vi "reward_behavior_michelle_visjitter_conswinAdapt_enticefx_TSLog_VF_fortraining_lightdetectionOG.vi"() -> ()   [LabVIEW 2019]
doc: "The myRIO Project template acquires acceleration data from the onboard accelerometer and displays the changes of acceleration values in a waveform chart."
uses:
  <vilib>/Analysis/Matrix/Datatypes/RealMatrix.ctl
  <vilib>/myRIO/Instrument Drivers/Onboard IO/DIO/typedefs/DIO Reference.ctl
  <vilib>/myRIO/Common/Instrument Driver Framework/Utilities/typedefs/myRIO Generic Hardware Reference.ctl
  <vilib>/myRIO/Common/Instrument Driver Framework/Utilities/typedefs/Hardware Version Enum.ctl
  <vilib>/myRIO/Common/Instrument Driver Framework/Utilities/typedefs/myRIO v1.0 Reference.ctl
  <vilib>/myRIO/Common/Instrument Driver Framework/Utilities/typedefs/Generic FPGA Reference.ctl
  <vilib>/myRIO/Common/Instrument Driver Framework/myRIO v1.0/DIO/typedefs/DIO Channels List.ctl
  <vilib>/myRIO/Common/Instrument Driver Framework/myRIO v1.0/DIO/typedefs/DIO Channels Enum.ctl
  <vilib>/userdefined/High Color/nirio_resource_hc.ctl
  <vilib>/myRIO/Common/Instrument Driver Framework/myRIO v1.0/Encoder/typedefs/Encoder Signal Mode.ctl
  <vilib>/myRIO/Instrument Drivers/Onboard IO/Encoder/typedefs/Encoder Reference.ctl
  <vilib>/myRIO/Common/Instrument Driver Framework/myRIO v1.0/Encoder/typedefs/Encoder Channels Enum.ctl
  <vilib>/myRIO/Common/Instrument Driver Framework/myRIO v1.0/Encoder/typedefs/Encoder Configuration v1.0.ctl
  <vilib>/myRIO/Instrument Drivers/Onboard IO/AI/typedefs/AI Reference.ctl
  <vilib>/myRIO/Common/Instrument Driver Framework/myRIO v1.0/AI/typedefs/AI Channels List.ctl
  <vilib>/myRIO/Common/Instrument Driver Framework/myRIO v1.0/AI/typedefs/AI Channels Enum.ctl
  <vilib>/myRIO/Common/Instrument Driver Framework/Utilities/typedefs/Analog Scaling Constants List.ctl
  <vilib>/myRIO/Common/Instrument Driver Framework/Utilities/typedefs/Analog Scaling Constants.ctl
  <vilib>/myRIO/Common/Instrument Driver Framework/Utilities/vis/Is FPGA Ref Available.vi
  <vilib>/myRIO/Common/Instrument Driver Framework/myRIO v1.0/DIO/vis/myRIO v1.1 Open DIO.vi
  <vilib>/myRIO/Instrument Drivers/Onboard IO/DIO/vis/Write.vi
  <vilib>/myRIO/Common/Instrument Driver Framework/myRIO v1.0/Encoder/vis/myRIO v1.1 Open Encoder.vi
  <vilib>/myRIO/Instrument Drivers/Onboard IO/Encoder/vis/Read.vi
  <vilib>/myRIO/Common/Instrument Driver Framework/myRIO v1.0/AI/vis/myRIO v1.1 Open AI.vi
  <vilib>/myRIO/Instrument Drivers/Onboard IO/AI/vis/Read.vi
  <vilib>/myRIO/Instrument Drivers/Onboard IO/DIO/vis/Read.vi
  <vilib>/myRIO/Common/Instrument Driver Framework/Utilities/vis/Validate Channels.vi
  <vilib>/myRIO/Common/Instrument Driver Framework/myRIO v1.0/DIO/vis/myRIO v1.0 Reserve DIO.vi
  <vilib>/myRIO/Common/Instrument Driver Framework/myRIO v1.0/Encoder/vis/myRIO v1.0 Reserve Encoder.vi
  <vilib>/myRIO/Common/Instrument Driver Framework/myRIO v1.0/AI/vis/myRIO v1.0 Reserve AI.vi
  <vilib>/myRIO/Common/Instrument Driver Framework/myRIO v1.0/Resource Manager/vis/myRIO v1.0 Reserve Channel List.vi
  <vilib>/myRIO/Common/Instrument Driver Framework/myRIO v1.0/DIO/vis/myRIO v1.0 Build MUX Configuration DIO.vi
  <vilib>/myRIO/Common/Instrument Driver Framework/myRIO v1.0/Encoder/vis/myRIO v1.0 Build MUX Configuration Encoder.vi
  <vilib>/myRIO/Common/Instrument Driver Framework/myRIO v1.0/AI/vis/myRIO v1.0 Build MUX Configuration AI.vi
  <vilib>/myRIO/Common/Instrument Driver Framework/myRIO v1.0/Resource Manager/vis/myRIO v1.0 Reserve Channel.vi
  <vilib>/myRIO/Common/Instrument Driver Framework/myRIO v1.0/Resource Manager/vis/myRIO v1.0 Unreserve Channel.vi
  <vilib>/myRIO/Common/Instrument Driver Framework/myRIO v1.0/Resource Manager/vis/myRIO v1.0 Create Configuration List.vi
  <vilib>/myRIO/Common/Instrument Driver Framework/myRIO v1.0/Resource Manager/vis/myRIO v1.0 Build Mutex Name.vi
  <vilib>/Utility/VariantDataType/GetNumericInfo.vi
  <vilib>/Utility/error.llb/Error Cluster From Error Code.vi
  <vilib>/myRIO/Common/Instrument Driver Framework/myRIO v1.0/myRIO v1.1 Open.vi
  <vilib>/myRIO/Common/Instrument Driver Framework/Utilities/vis/IO Manager.vi
  <vilib>/myRIO/Common/Instrument Driver Framework/Utilities/vis/Configuration Manager.vi
  <vilib>/myRIO/Common/Instrument Driver Framework/myRIO v1.0/Resource Manager/vis/myRIO v1.0 Configure IO.vi
  <vilib>/myRIO/Common/Instrument Driver Framework/myRIO v1.0/myRIO v1.0 Close.vi
  <vilib>/myRIO/Common/Instrument Driver Framework/myRIO v1.0/Encoder/vis/myRIO v1.0 Configure Encoder.vi
  <vilib>/myRIO/Common/Instrument Driver Framework/myRIO v1.0/Encoder/vis/myRIO v1.0 Read Encoder.vi
  <vilib>/myRIO/Common/Instrument Driver Framework/myRIO v1.0/DIO/vis/myRIO v1.0 Write DIO.vi
  <vilib>/myRIO/Common/Instrument Driver Framework/myRIO v1.0/DIO/vis/myRIO v1.0 Read DIO.vi
  <vilib>/myRIO/Common/Instrument Driver Framework/myRIO v1.0/AI/vis/myRIO v1.0 Get Scaling Constants AI.vi
  <vilib>/myRIO/Common/Instrument Driver Framework/myRIO v1.0/AI/vis/myRIO v1.0 Read AI.vi
  <vilib>/myRIO/Express VI/Onboard IO/Encoder/Encoder Express VI.xnode
  <vilib>/myRIO/Instrument Drivers/Onboard IO/Encoder/vis/myRIO Encoder Open.xnode
  <vilib>/myRIO/Common/Instrument Driver Framework/myRIO v1.0/Encoder/typedefs/Encoder Count Direction Enum.ctl
  <vilib>/myRIO/Express VI/Onboard IO/DO/DO Express VI.xnode
  <vilib>/myRIO/Instrument Drivers/Onboard IO/DIO/vis/myRIO DIO Open.xnode
  <vilib>/myRIO/Express VI/Onboard IO/DI/DI Express VI.xnode
  <vilib>/myRIO/Express VI/Onboard IO/AI/AI Express VI.xnode
  <vilib>/myRIO/Instrument Drivers/Onboard IO/AI/vis/myRIO AI Open.xnode
  <vilib>/myRIO/Instrument Drivers/Onboard IO/Encoder/Encoder.lvlib
  <vilib>/myRIO/Instrument Drivers/Onboard IO/DIO/DIO.lvlib
  <vilib>/myRIO/Instrument Drivers/Onboard IO/AI/AI.lvlib
  <vilib>/Analysis/Matrix/NI_Matrix.lvlib
panel:
  out "Light":dbl
  out "LightPlot":dbl[](graph)
  out "LightArray":dbl[](array[numeric])
  out "AutoEnticeLimit":i32=1000
  out "GetVidFrame":i32
  out "VidTS":dbl[][](array[numeric])
  out "VidFrameClock":i32
  out "EntTS":dbl[][](array[numeric])
  out "TimeLag":dbl
  out "Lag2":dbl
  out "TestTime":dbl
  out "RewTS":dbl[][](array[numeric])
  out "ConsTS":dbl[][](array[numeric])
  out "LickTS":dbl[][](array[numeric])
  out "ContrastChoice":dbl
  out "Its":i32
  out "BurstCriteria":dbl
  out "LickBurst 2":bool
  out "LickBurst":bool
  out "Enticements":i32
  in  "Entice":bool
  out "Misses":i32
  out "GoAhead":bool
  out "TimeOutDuration":i32
  out "ActiveTime":dbl
  out "ConsumptionGo":bool=TRUE
  out "Consumption_Period":i32
  out "Watch_Display":bool=TRUE
  in  "Give reward":bool
  out "Timings":dbl[](array[numeric])
  out "ISI":dbl
  out "ISI start time":dbl
  out "Time_out":bool=TRUE
  out "Time since lick":dbl
  out "Time of last lick":dbl
  out "Rewarded trials":dbl[](array[numeric])
  out "Rewards":u16
  out "Active Trial":bool
  out "Array temp2":T1
  out "Stimuli Loaded":bool
  out "Stim_ID":dbl[](array[numeric])
  out "Reward_mat":dbl[](array[numeric])
  out "Reward":bool=TRUE
  out "Frame clock":i32
  out "Licks":u32
  out "Lick":bool
  out "Time":dbl
  out "Stop":bool
  in  "Frames to collect":u32
  out "Overflow?":bool
  out "Counter Value":i32
  out "Velocity":dbl
  out "Velocity Plot":dbl[](graph)
  out "Velocity array":dbl[](array[numeric])
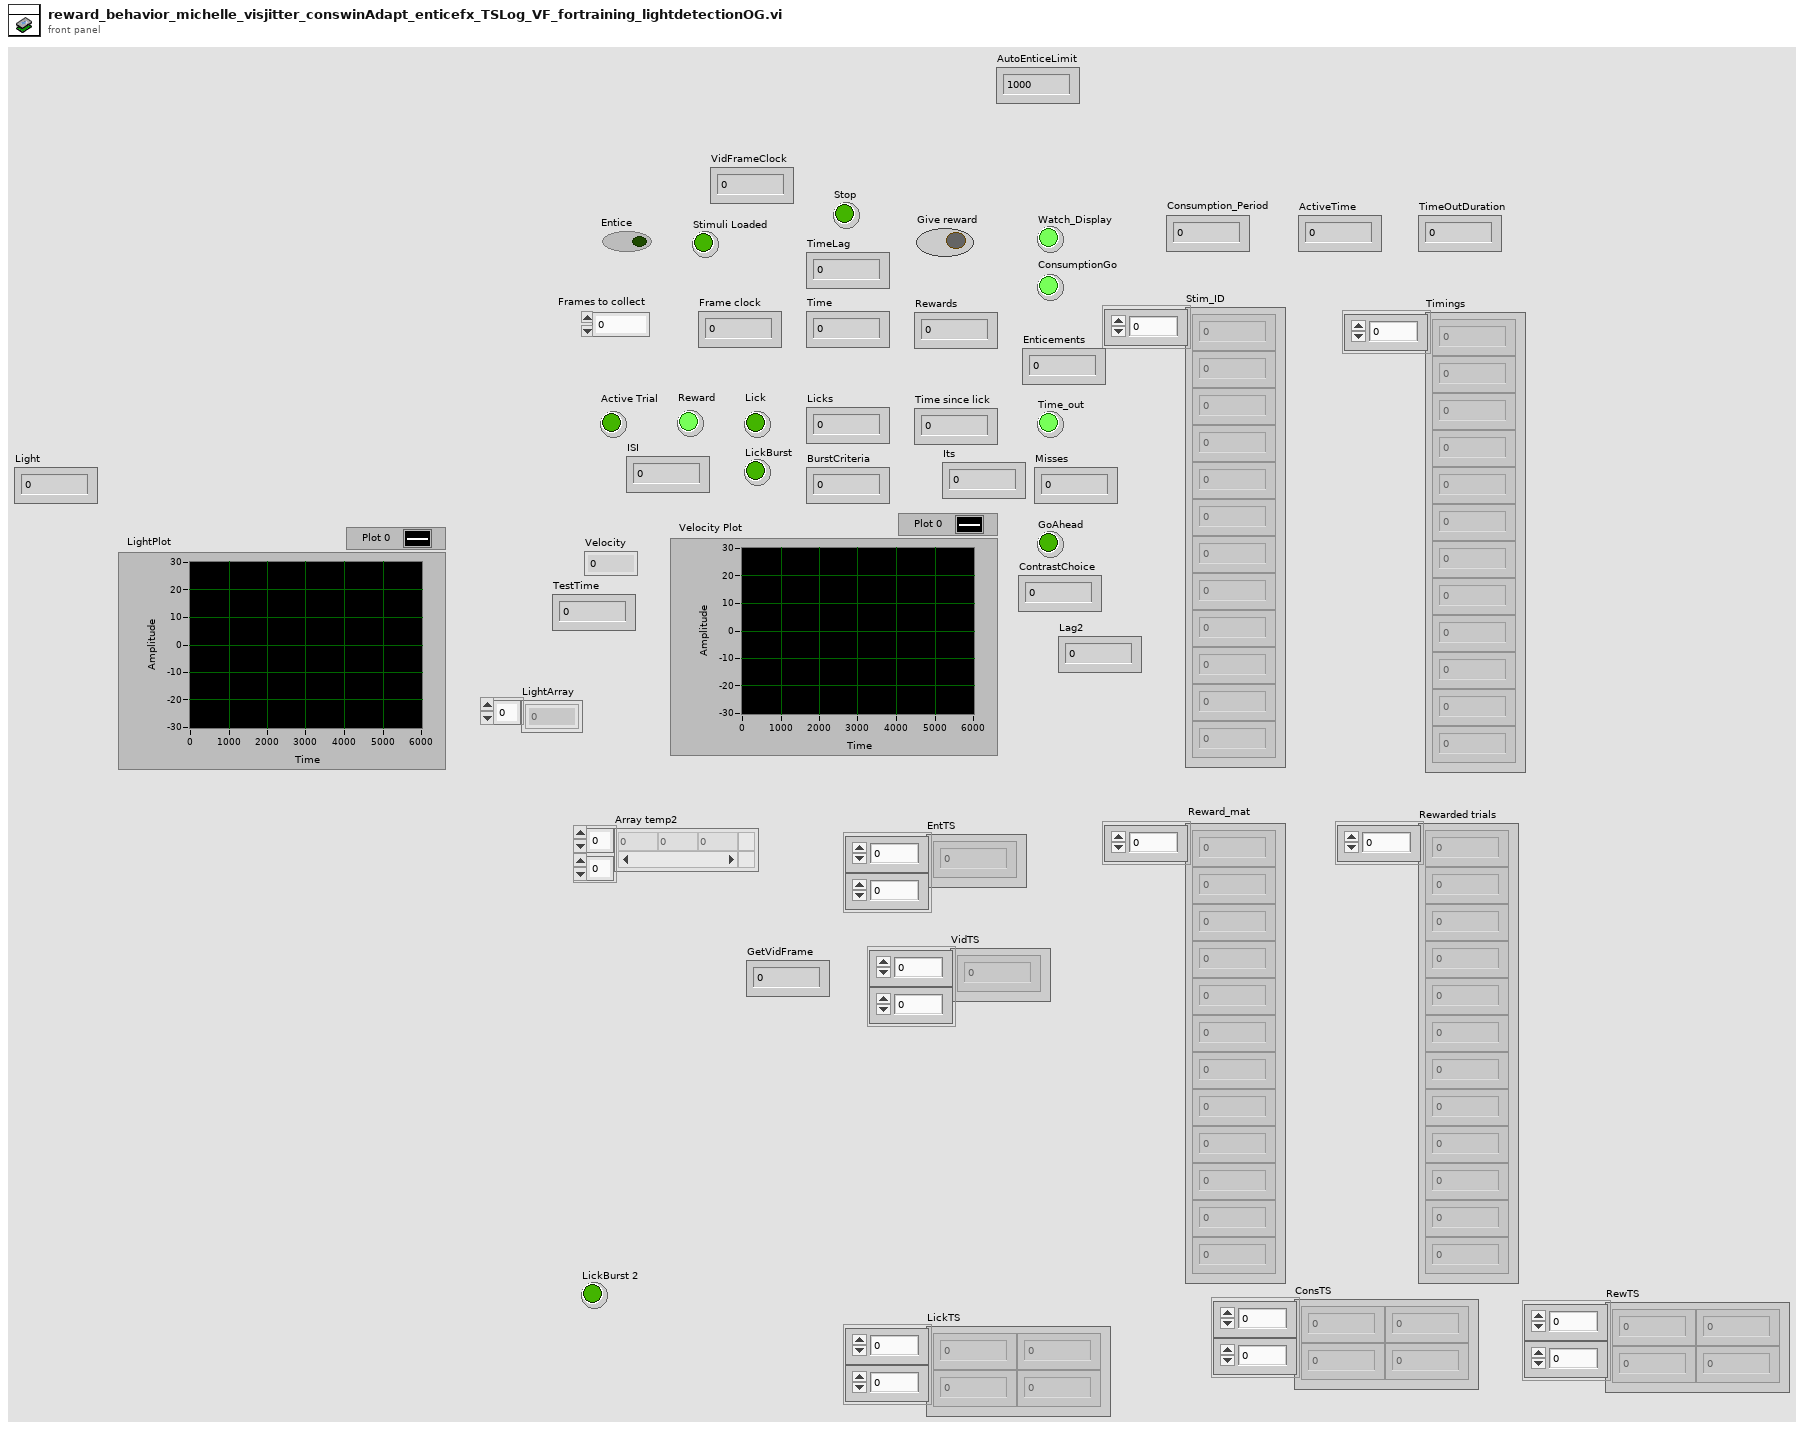
[diagram p1: front panel]
types:
  T1 = typedef "NI_Matrix.lvlib/RealMatrix.ctl" = dbl[][]
  T2 = typedef "DIO.lvlib/DIO Reference.ctl" = cluster{"myRIO Reference":T3, "DIO Channels List":T7}
  T3 = typedef "myRIO Generic Hardware Reference.ctl" = cluster{"myRIO Model":T4, "myRIO Hardware Reference":T5}
  T4 = typedef "Hardware Version Enum.ctl" = enum16{"Unknown", "myRIO-1900", "myRIO-1950", "roboRIO", "NI ELVIS RIO CM", "ELVIS III"}
  T5 = typedef "myRIO v1.0 Reference.ctl" = cluster{"Generic FPGA Reference":T6, "Allow multiple opens":bool}
  T6 = typedef "Generic FPGA Reference.ctl" = refnum<k20>
  T7 = typedef "DIO Channels List.ctl" = T8[]
  T8 = typedef "DIO Channels Enum.ctl" = enum16{"Not Connected", "C/DIO0", "C/DIO1", "C/DIO2", "C/DIO3", "C/DIO4", "C/DIO5", "C/DIO6", "C/DIO7", "A/DIO0", "A/DIO1", "A/DIO2", "A/DIO3", "A/DIO4", "A/DIO5", "A/DIO6", "A/DIO7", "A/DIO8", "A/DIO9", "A/DIO10", "A/DIO11", "A/DIO12", "A/DIO13", "A/DIO14", "A/DIO15", "A/DIO16", "A/DIO17", "A/DIO18", "A/DIO19", "B/DIO0", "B/DIO1", "B/DIO2", "B/DIO3", "B/DIO4", "B/DIO5", "B/DIO6", "B/DIO7", "B/DIO8", "B/DIO9", "B/DIO10", "B/DIO11", "B/DIO12", "B/DIO13", "B/DIO14", "B/DIO15", "B/DIO16", "B/DIO17", "B/DIO18", "B/DIO19", "LED0", "LED1", "LED2", "LED3", "Button0", "DIO/DIO0", "DIO/DIO1", "DIO/DIO2", "DIO/DIO3", "DIO/DIO4", "DIO/DIO5", "DIO/DIO6", "DIO/DIO7", "DIO/DIO8", "DIO/DIO9", "SPI/CS0", "SPI/CS1", "SPI/CS2", "SPI/CS3", "LED RADIO (Green)", "LED RADIO (Red)", "LED COMM (Green)", "LED COMM (Red)", "LED MODE (Green)", "LED MODE (Red)"}
  T9 = typedef "nirio_resource_hc.ctl" = tag
  T10 = typedef "Encoder.lvlib/Encoder Reference.ctl" = cluster{"myRIO Reference":T3, "Encoder Channels Enum":T11}
  T11 = typedef "Encoder Channels Enum.ctl" = enum16{"Not Connected", "C/ENC0", "C/ENC1", "A/ENC", "A/ENC0", "A/ENC1", "A/ENC2", "A/ENC3", "A/ENC4", "A/ENC5", "A/ENC6", "A/ENC7", "A/ENC8", "A/ENC9", "B/ENC", "B/ENC0", "B/ENC1", "B/ENC2", "B/ENC3", "B/ENC4", "B/ENC5", "B/ENC6", "B/ENC7", "B/ENC8", "B/ENC9", "DIO/ENC0", "DIO/ENC1", "DIO/ENC2", "DIO/ENC3", "DIO/ENC4"}
  T12 = typedef "Encoder Signal Mode.ctl" = enum16{"Quadrature phase signal", "Step and direction signal"}
  T13 = typedef "AI.lvlib/AI Reference.ctl" = cluster{"myRIO Reference":T3, "AI Channels List":T14, "AI Scaling Constants List":T16}
  T14 = typedef "AI Channels List.ctl" = T15[]
  T15 = typedef "AI Channels Enum.ctl" = enum16{"Not Connected", "AudioIn/Left", "AudioIn/Right", "C/AI0", "C/AI1", "A/AI0", "A/AI1", "A/AI2", "A/AI3", "A/AI4", "A/AI5", "A/AI6", "A/AI7", "B/AI0", "B/AI1", "B/AI2", "B/AI3", "B/AI4", "B/AI5", "B/AI6", "B/AI7", "AI/AI0", "AI/AI1", "AI/AI2", "AI/AI3", "A/AI0 (DIFF)", "A/AI1 (DIFF)", "A/AI2 (DIFF)", "A/AI3 (DIFF)", "B/AI0 (DIFF)", "B/AI1 (DIFF)", "B/AI2 (DIFF)", "B/AI3 (DIFF)"}
  T16 = typedef "Analog Scaling Constants List.ctl" = T17[]
  T17 = typedef "Analog Scaling Constants.ctl" = cluster{"LSB Weight (Volts)":dbl, "Offset (Volts)":dbl, "Signed?":bool}
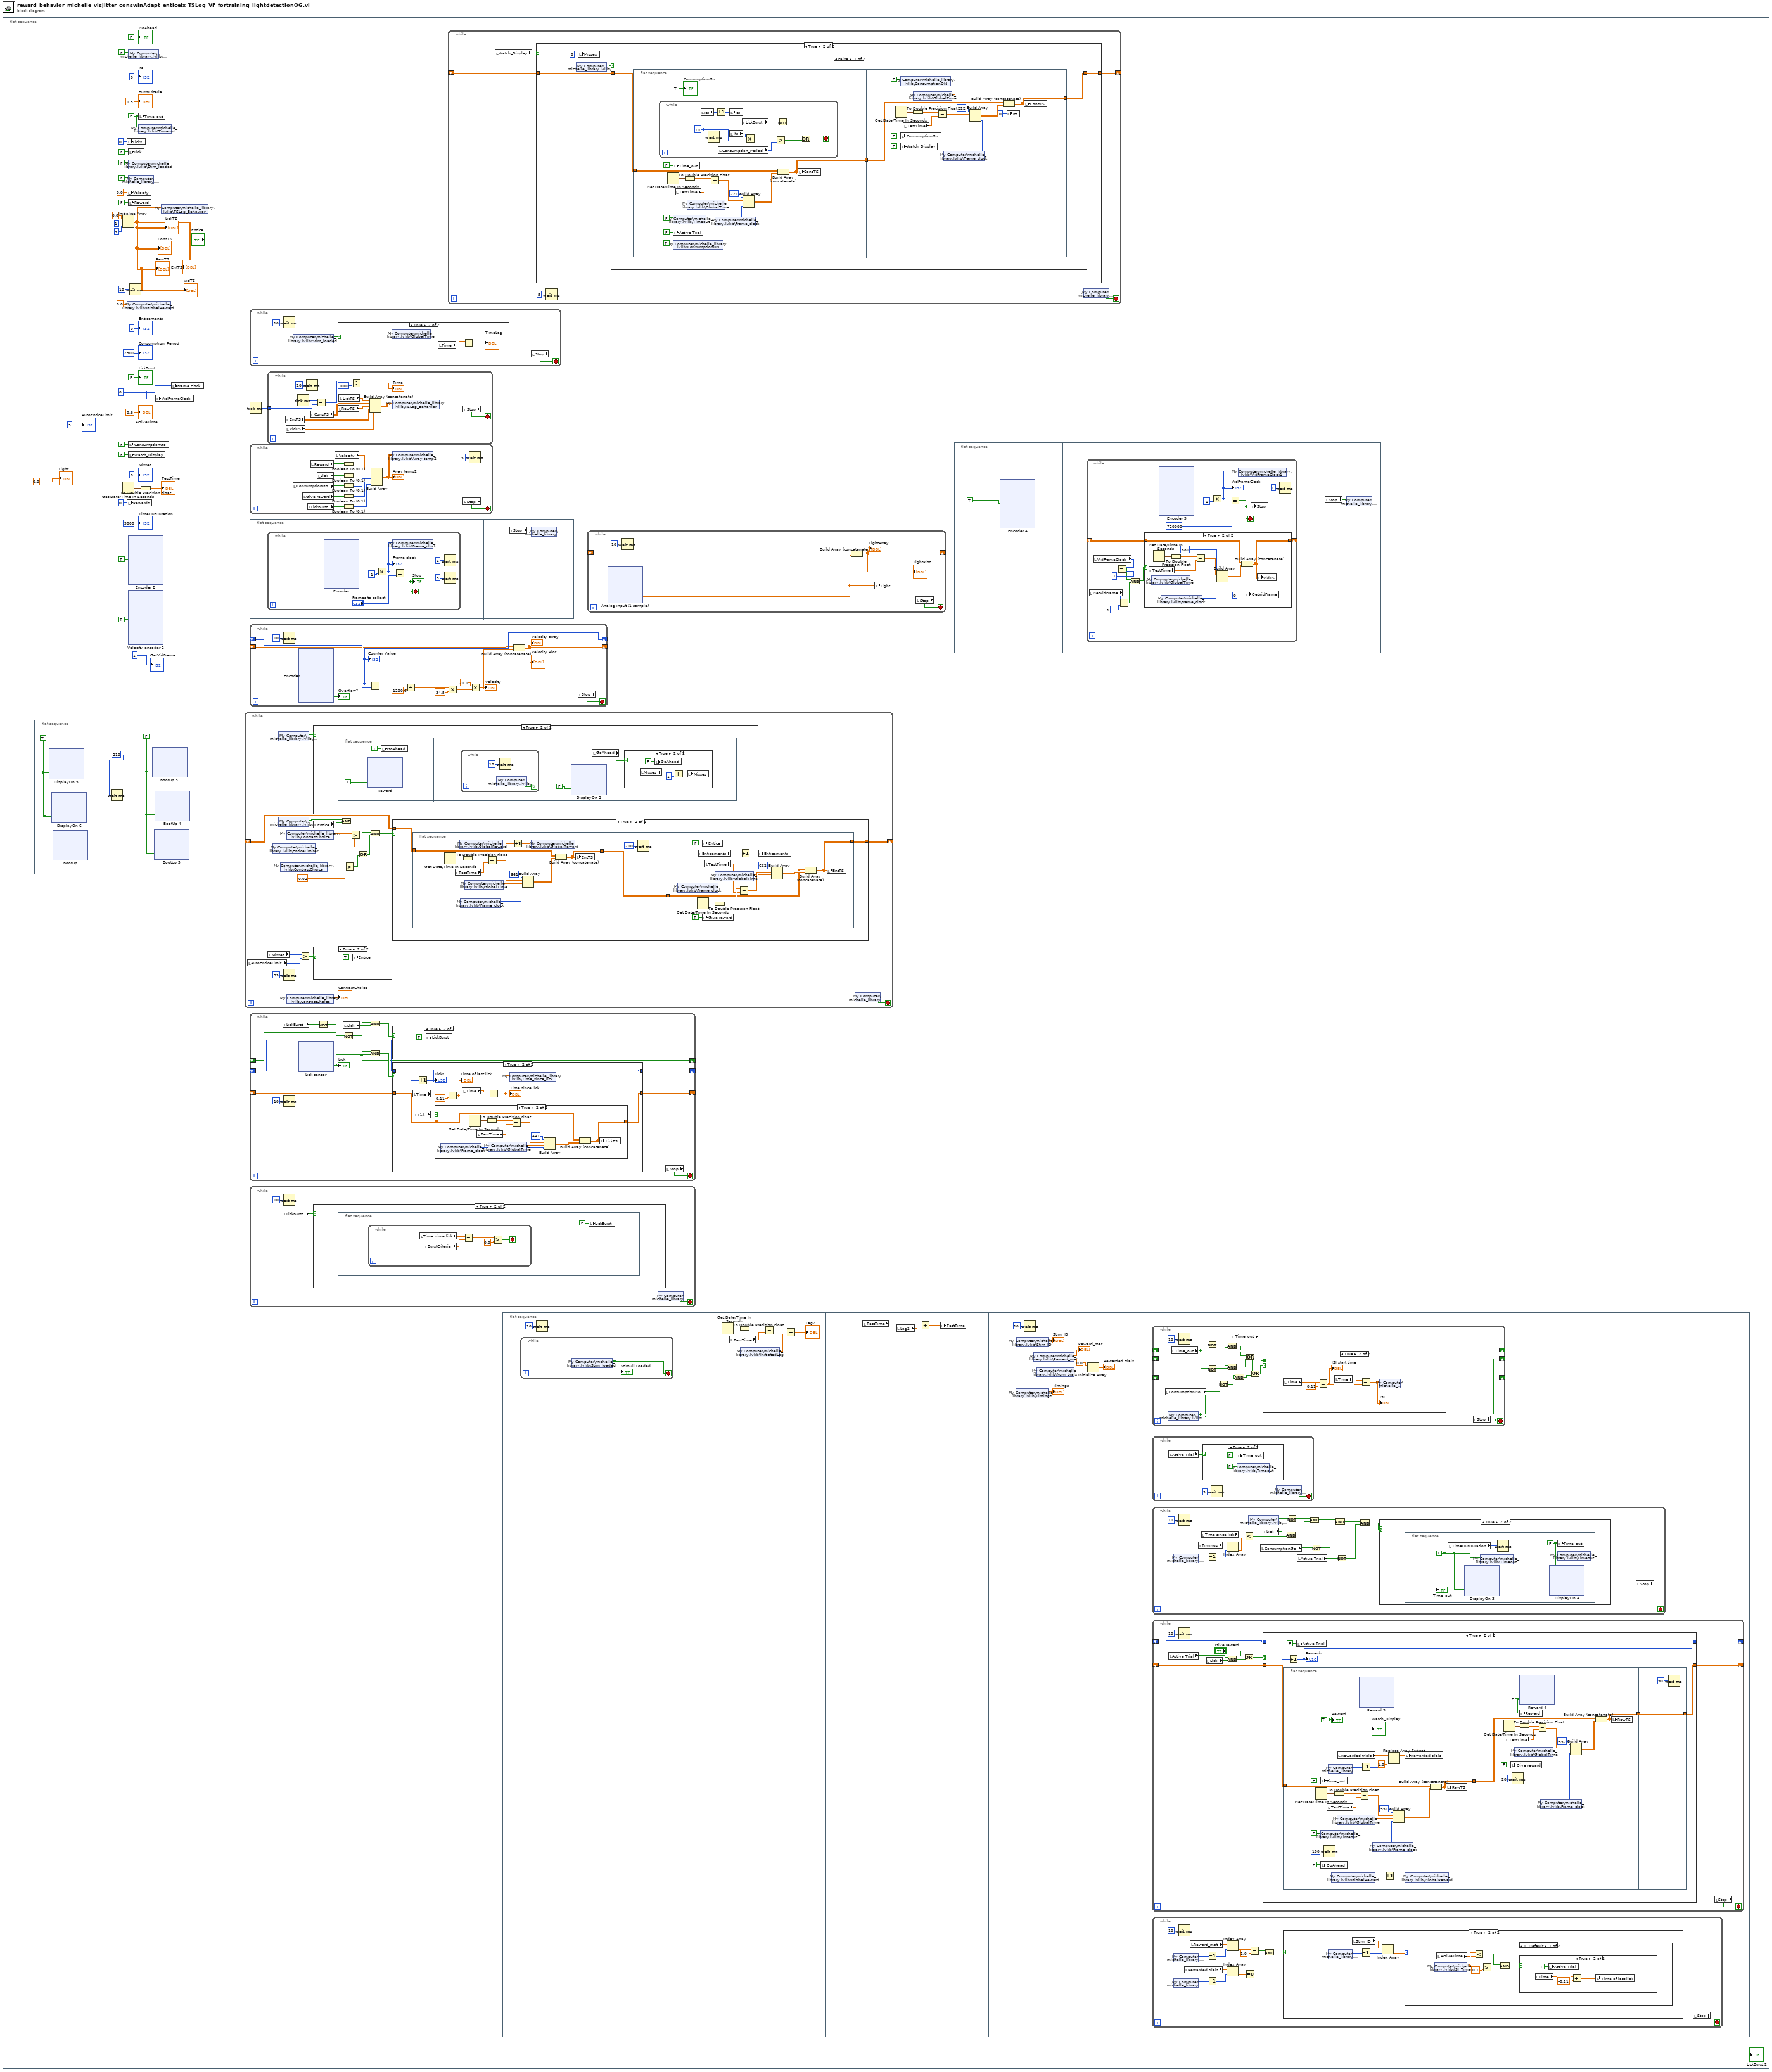
[diagram p0: block diagram]
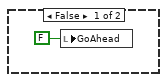
[diagram p7: hidden frame]
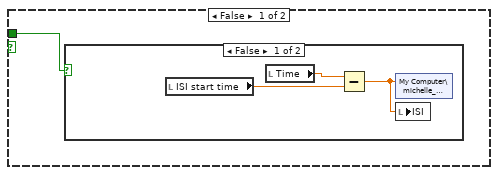
[diagram p13: hidden frame]
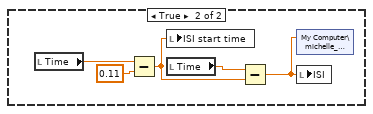
[diagram p14: hidden frame]
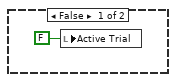
[diagram p15: hidden frame]
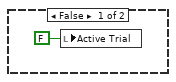
[diagram p16: hidden frame]
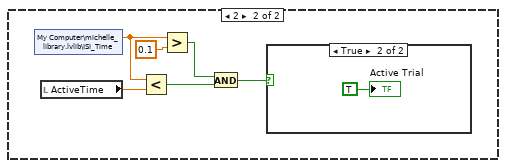
[diagram p17: hidden frame]
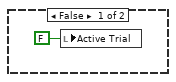
[diagram p18: hidden frame]
diagram:
  n1 = flat-sequence {
    frame #0 {
      w23 = FALSE ("Time_out")
      w5 = u32 0 ("Frames")
      n2 = flat-sequence {
        frame #0 {
          w35 = TRUE
          n3 = xnode "DisplayOn 5"("C/DIO2 (DIO2)"=w35) -> ()  [unwired: 1 in, 1 out]
          n4 = xnode "DisplayOn 6"("C/DIO1 (DIO1)"=w35) -> ()  [unwired: 1 in, 1 out]
          n5 = xnode "BootUp"("C/DIO3 (DIO3)"=w35) -> ()  [unwired: 1 in, 1 out]
        }
        frame #1 {
          n6 = Wait (ms)(milliseconds to wait=210) -> ()  [unwired: 1 out]
        }
        frame #2 {
          w142 = FALSE
          n7 = xnode "BootUp 3"("C/DIO2 (DIO2)"=w142) -> ()  [unwired: 1 in, 1 out]
          n8 = xnode "BootUp 5"("C/DIO3 (DIO3)"=w142) -> ()  [unwired: 1 in, 1 out]
          n9 = xnode "BootUp 4"("C/DIO1 (DIO1)"=w142) -> ()  [unwired: 1 in, 1 out]
        }
      }
      n10 = Get Date/Time In Seconds() -> (seconds since 1Jan1904=w7:timestamp)
      n11 = Initialize Array(0.0, 1, 3) -> (w4:dbl[][])
      "LickTS" <- w4
      "ConsTS" <- w4
      "RewTS" <- w4
      "EntTS" <- w4
      "VidTS" <- w4
      n12 = local write "Licks"(u32 0 ("Licks")) -> ()
      n13 = local write "Velocity"(0.0 ("Velocity")) -> ()
      n14 = shared-variable "My Computer\\michelle_library.lvlib\\GlobalReward"(0.0) -> ()  [unwired: 1 in, 1 out]
      n15 = local write "Rewards"(u16 0 ("Rewards")) -> ()
      n16 = shared-variable "My Computer\\michelle_library.lvlib\\Display"(FALSE ("Display")) -> ()  [unwired: 1 in, 1 out]
      n17 = local write "Lick"(FALSE ("Lick")) -> ()
      n18 = shared-variable "My Computer\\michelle_library.lvlib\\Stim_loaded"(FALSE ("Stim_loaded")) -> ()  [unwired: 1 in, 1 out]
      n19 = shared-variable "My Computer\\michelle_library.lvlib\\Stop"(FALSE ("Stop")) -> ()  [unwired: 1 in, 1 out]
      n20 = local write "Reward"(FALSE ("Give reward")) -> ()
      n21 = local write "ConsumptionGo"(FALSE ("ConsumptionGo")) -> ()
      n22 = local write "Watch_Display"(FALSE ("Watch_Display")) -> ()
      n23 = xnode "Encoder 2"("Reset Counter"=TRUE) -> ()  [unwired: 1 in, 4 out]
      n24 = xnode "Velocity encoder 2"("Reset Counter"=TRUE) -> ()  [unwired: 1 in, 4 out]
      n25 = Wait (ms)(milliseconds to wait=u32 10) -> ()  [unwired: 1 out]
      n26 = local write "Time_out"(w23) -> ()
      n27 = shared-variable "My Computer\\michelle_library.lvlib\\Timeout"(w23) -> ()  [unwired: 1 in, 1 out]
      n28 = To Double Precision Float(number=w7) -> (double precision float=→"TestTime":dbl)
      n29 = local write "VidFrameClock"(w5) -> ()
      n30 = shared-variable "My Computer\\michelle_library.lvlib\\TSLog_Behavior"(w4) -> ()  [unwired: 1 in, 1 out]
      n31 = local write "Frame clock"(w5) -> ()
      "Consumption_Period" <- 2500
      "ActiveTime" <- 0.6
      "TimeOutDuration" <- 3000
      "GoAhead" <- FALSE
      "Misses" <- 0
      "Enticements" <- 0
      "LickBurst" <- FALSE
      "BurstCriteria" <- 0.5
      "Its" <- 0
      "GetVidFrame" <- 1
      "AutoEnticeLimit" <- 5
      "Light" <- 0.0
    }
    frame #1 {
      n32 = while {
        shift-right: [w527] -> _
        shift-left: _ -> [w528]
        stop <- w538 stop-if-true
        n33 = local read "AutoEnticeLimit"() -> (w519:i32)
        n34 = local read "Misses"() -> (w520:i32)
        n35 = shared-variable "My Computer\\michelle_library.lvlib\\EnticeLimiter"() -> (w526:dbl)  [unwired: 1 in, 1 out]
        n36 = shared-variable "My Computer\\michelle_library.lvlib\\Display"() -> (w537:bool)  [unwired: 1 in, 1 out]
        n37 = shared-variable "My Computer\\michelle_library.lvlib\\Display"() -> (w535:bool)  [unwired: 1 in, 1 out]
        n38 = shared-variable "My Computer\\michelle_library.lvlib\\ContrastChoice"() -> (w522:dbl)  [unwired: 1 in, 1 out]
        n39 = Wait (ms)(milliseconds to wait=35) -> ()  [unwired: 1 out]
        n40 = shared-variable "My Computer\\michelle_library.lvlib\\ContrastChoice"() -> (w531:dbl)  [unwired: 1 in, 1 out]
        n41 = shared-variable "My Computer\\michelle_library.lvlib\\ContrastChoice"() -> (→"ContrastChoice":dbl)  [unwired: 1 in, 1 out]
        n42 = Greater?(x=w520, y=w519) -> (0:w536:bool)
        n43 = case shown="True" w537 {
          frame False {
            n44 = local write "GoAhead"(FALSE) -> ()
          }
          frame True {
            n45 = flat-sequence {
              frame #0 {
                n46 = xnode "Reward"("C/DIO2 (DIO2)"=TRUE) -> ()  [unwired: 1 in, 1 out]
                n47 = local write "GoAhead"(TRUE) -> ()
              }
              frame #1 {
                n48 = while {
                  stop <- w612 continue-if-true
                  n49 = shared-variable "My Computer\\michelle_library.lvlib\\Display"() -> (w612:bool)  [unwired: 1 in, 1 out]
                  n50 = Wait (ms)(milliseconds to wait=10) -> ()  [unwired: 1 out]
                }
              }
              frame #2 {
                n51 = xnode "DisplayOn 2"("C/DIO2 (DIO2)"=FALSE) -> ()  [unwired: 1 in, 1 out]
                n52 = local read "GoAhead"() -> (w614:bool)
                n53 = case shown="True" w614 {
                  frame False {
                  }
                  frame True {
                    n54 = local read "Misses"() -> (w653:i32)
                    n55 = local write "GoAhead"(FALSE) -> ()
                    n56 = Add(x=w653, y=1) -> (x+y=w651:i32)
                    n57 = local write "Misses"(w651) -> ()
                  }
                }
              }
            }
          }
        }
        n58 = local read "Entice"() -> (w534:bool)
        n59 = case shown="True" w536 {
          frame False {
          }
          frame True {
            n60 = local write "Entice"(TRUE) -> ()
          }
        }
        n61 = And(x=w535, y=w534) -> (x .and. y?=w532:bool)
        n62 = Greater?(x=w522, y=0.02) -> (0:w523:bool)
        n63 = Greater?(x=w531, y=w526) -> (0:w524:bool)
        n64 = Or(x=w524, y=w523) -> (x .or. y?=w525:bool)
        n65 = And(x=w532, y=w525) -> (x .and. y?=w530:bool)
        n66 = case shown="True" w530 {
          tunnel: w528 -> [w539 w543]
          tunnel: [w539 w540] -> w527
          frame False {
          }
          frame True {
            n67 = flat-sequence {
              tunnel: w543 -> [w546]
              tunnel: [w545] -> w542
              tunnel: w542 -> [w556]
              tunnel: [w556] -> w541
              tunnel: w541 -> [w560]
              tunnel: [w559] -> w540
              frame #0 {
                n68 = Get Date/Time In Seconds() -> (seconds since 1Jan1904=w553:timestamp)
                n69 = local read "TestTime"() -> (w548:dbl)
                n70 = shared-variable "My Computer\\michelle_library.lvlib\\GlobalReward"() -> (w555:dbl)  [unwired: 1 in, 1 out]
                n71 = shared-variable "My Computer\\michelle_library.lvlib\\Frame_clock"() -> (w544:u32)  [unwired: 1 in, 1 out]
                n72 = To Double Precision Float(number=w553) -> (double precision float=w552:dbl)
                n73 = shared-variable "My Computer\\michelle_library.lvlib\\GlobalTime"() -> (w547:dbl)  [unwired: 1 in, 1 out]
                n74 = Subtract(x=w552, y=w548) -> (x-y=w551:dbl)
                n75 = Increment(x=w555) -> (x+1=w554:dbl)
                n76 = Build Array(661, w551, w547, w544) -> (w550:T1)
                n77 = shared-variable "My Computer\\michelle_library.lvlib\\GlobalReward"(w554) -> ()  [unwired: 1 in, 1 out]
                n78 = Build Array (concatenate) ("Build Matrix")(w546, w550) -> (w545:T1)
                n79 = local write "EntTS"(w545) -> ()
              }
              frame #1 {
                n80 = Wait (ms)(milliseconds to wait=200) -> ()  [unwired: 1 out]
              }
              frame #2 {
                n81 = shared-variable "My Computer\\michelle_library.lvlib\\Frame_clock"() -> (w558:u32)  [unwired: 1 in, 1 out]
                n82 = Get Date/Time In Seconds() -> (seconds since 1Jan1904=w567:timestamp)
                n83 = local read "Enticements"() -> (w569:i32)
                n84 = local write "Entice"(FALSE) -> ()
                n85 = local write "Give reward"(TRUE) -> ()
                n86 = local read "TestTime"() -> (w561:dbl)
                n87 = To Double Precision Float(number=w567) -> (double precision float=w566:dbl)
                n88 = shared-variable "My Computer\\michelle_library.lvlib\\GlobalTime"() -> (w562:dbl)  [unwired: 1 in, 1 out]
                n89 = Subtract(x=w566, y=w561) -> (x-y=w565:dbl)
                n90 = Increment(x=w569) -> (x+1=w568:i32)
                n91 = local write "Enticements"(w568) -> ()
                n92 = Build Array(662, w565, w562, w558) -> (w564:T1)
                n93 = Build Array (concatenate) ("Build Matrix")(w560, w564) -> (w559:T1)
                n94 = local write "EntTS"(w559) -> ()
              }
            }
          }
        }
        n95 = shared-variable "My Computer\\michelle_library.lvlib\\Stop"() -> (w538:bool)  [unwired: 1 in, 1 out]
      }
      n96 = while {
        stop <- w505 stop-if-true
        n97 = Wait (ms)(milliseconds to wait=u32 10) -> ()  [unwired: 1 out]
        n98 = shared-variable "My Computer\\michelle_library.lvlib\\Stim_loaded"() -> (w506:bool)  [unwired: 1 in, 1 out]
        n99 = case shown="True" w506 {
          frame False {
          }
          frame True {
            n100 = shared-variable "My Computer\\michelle_library.lvlib\\GlobalTime"() -> (w507:dbl)  [unwired: 1 in, 1 out]
            n101 = local read "Time"() -> (w508:dbl)
            n102 = Subtract(x=w507, y=w508) -> (x-y=→"TimeLag":dbl)
          }
        }
        n103 = local read "Stop"() -> (w505:bool)
      }
      n104 = Tick Count (ms)() -> (millisecond timer value=w340:u32)
      n105 = while {
        stop <- w714 stop-if-true
        n106 = local read "ConsumptionGo"() -> (w712:bool)
        n107 = local read "Give reward"() -> (w711:bool)
        n108 = local read "LickBurst"() -> (w708:bool)
        n109 = local read "Reward"() -> (w719:bool)
        n110 = local read "Lick"() -> (w720:bool)
        n111 = local read "Velocity"() -> (w718:dbl)
        n112 = Boolean To (0,1)(Boolean=w719) -> (0, 1=w717:i16)
        n113 = Boolean To (0,1)(Boolean=w720) -> (0, 1=w716:i16)
        n114 = Boolean To (0,1)(Boolean=w712) -> (0, 1=w710:i16)
        n115 = Boolean To (0,1)(Boolean=w711) -> (0, 1=w709:i16)
        n116 = Boolean To (0,1)(Boolean=w708) -> (0, 1=w707:i16)
        n117 = Build Array(w718, w717, w716, w710, w709, w707) -> (w713:T1)
        "Array temp2" <- w713
        n118 = shared-variable "My Computer\\michelle_library.lvlib\\Array temp2"(w713) -> ()  [unwired: 1 in, 1 out]
        n119 = local read "Stop"() -> (w714:bool)
        n120 = Wait (ms)(milliseconds to wait=u32 5) -> ()  [unwired: 1 out]
      }
      n121 = flat-sequence {
        frame #0 {
          n122 = while {
            stop <- w1033 stop-if-true
            n123 = xnode "Encoder"() -> ("Counter Value"=w1037:i32)  [unwired: 2 in, 3 out]
            n124 = Multiply(x=w1037, y=-1) -> (x*y=w1032:i32)
            "Frame clock" <- w1032
            n125 = shared-variable "My Computer\\michelle_library.lvlib\\Frame_clock"(w1032) -> ()  [unwired: 1 in, 1 out]
            n126 = Equal?(x=w1032, y="Frames to collect") -> (x = y?=w1033:bool)
            "Stop" <- w1033
            n127 = Wait (ms)(milliseconds to wait=u32 1) -> ()  [unwired: 1 out]
            n128 = Wait (ms)(milliseconds to wait=u32 5) -> ()  [unwired: 1 out]
          }
        }
        frame #1 {
          n129 = local read "Stop"() -> (w1085:bool)
          n130 = shared-variable "My Computer\\michelle_library.lvlib\\Stop"(w1085) -> ()  [unwired: 1 in, 1 out]
        }
      }
      n131 = while {
        shift-right: [w1172] -> _
        shift-left: _ -> [w1173]
        shift-right: [w1164] -> _
        shift-left: _ -> [w1163]
        stop <- w1162 stop-if-true
        n132 = Wait (ms)(milliseconds to wait=u32 10) -> ()  [unwired: 1 out]
        n133 = xnode "Encoder"() -> ("Counter Value"=w1172:i32, "Overflow?"=→"Overflow?":bool)  [unwired: 2 in, 2 out]
        "Counter Value" <- w1172
        n134 = Subtract(x=w1172, y=w1173) -> (x-y=w1165:i32)
        n135 = Divide(x=w1165, y=1200.0 ("600")) -> (x/y=w1170:dbl)
        n136 = Multiply(x=w1170, y=34.5) -> (x*y=w1168:dbl)
        n137 = Multiply(x=20.0, y=w1168) -> (x*y=w1166:dbl)
        "Velocity" <- w1166
        n138 = Build Array (concatenate)(w1163, w1166) -> (w1164:dbl[])
        "Velocity Plot" <- w1164
        "Velocity array" <- w1164
        n139 = local read "Stop"() -> (w1162:bool)
      }
      n140 = while {
        shift-right: [w1098] -> _
        shift-left: _ -> [w1097]
        shift-right: [w1092] -> _
        shift-left: _ -> [w1095]
        shift-right: [w1086] -> _
        shift-left: _ -> [w1087]
        stop <- w1096 stop-if-true
        n141 = local read "LickBurst"() -> (w1089:bool)
        n142 = Wait (ms)(milliseconds to wait=u32 10) -> ()  [unwired: 1 out]
        n143 = xnode "Lick sensor"() -> ("C/DIO1 (DIO1)"=w1092:bool)  [unwired: 1 in, 1 out]
        "Lick" <- w1092
        n144 = Not(x=w1089) -> (.not. x?=w1088:bool)
        n145 = Not(x=w1095) -> (.not. x?=w1094:bool)
        n146 = local read "Lick"() -> (w1090:bool)
        n147 = And(x=w1088, y=w1090) -> (x .and. y?=w1091:bool)
        n148 = And(x=w1094, y=w1092) -> (x .and. y?=w1093:bool)
        n149 = case shown="True" w1091 {
          frame False {
          }
          frame True {
            n150 = local write "LickBurst"(TRUE) -> ()
          }
        }
        n151 = case shown="True" w1093 {
          tunnel: [w1105 w1115] -> w1098
          tunnel: w1097 -> [w1105 w1114]
          tunnel: w1087 -> [w1101 w1106]
          tunnel: [w1101 w1108] -> w1086
          frame False {
            n152 = local read "Time of last lick"() -> (w1103:dbl)
            n153 = local read "Time"() -> (w1104:dbl)
            n154 = Subtract(x=w1104, y=w1103) -> (x-y=w1102:dbl)
            n155 = shared-variable "My Computer\\michelle_library.lvlib\\Time_since_lick"(w1102) -> ()  [unwired: 1 in, 1 out]
            n156 = local write "Time since lick"(w1102) -> ()
          }
          frame True {
            n157 = local read "Time"() -> (w1111:dbl)
            n158 = local read "Lick"() -> (w1107:bool)
            n159 = Increment(x=w1114) -> (x+1=w1115:u32)
            "Licks" <- w1115
            n160 = case shown="True" w1107 {
              tunnel: w1106 -> [w1116 w1122]
              tunnel: [w1116 w1121] -> w1108
              frame False {
              }
              frame True {
                n161 = shared-variable "My Computer\\michelle_library.lvlib\\Frame_clock"() -> (w1117:u32)  [unwired: 1 in, 1 out]
                n162 = Get Date/Time In Seconds() -> (seconds since 1Jan1904=w1124:timestamp)
                n163 = local read "TestTime"() -> (w1119:dbl)
                n164 = To Double Precision Float(number=w1124) -> (double precision float=w1120:dbl)
                n165 = shared-variable "My Computer\\michelle_library.lvlib\\GlobalTime"() -> (w1118:dbl)  [unwired: 1 in, 1 out]
                n166 = Subtract(x=w1120, y=w1119) -> (x-y=w1125:dbl)
                n167 = Build Array(441, w1125, w1118, w1117) -> (w1126:T1)
                n168 = Build Array (concatenate) ("Build Matrix")(w1122, w1126) -> (w1121:T1)
                n169 = local write "LickTS"(w1121) -> ()
              }
            }
            n170 = Subtract(x=w1111, y=0.11) -> (x-y=w1109:dbl)
            "Time of last lick" <- w1109
            n171 = local read "Time"() -> (w1113:dbl)
            n172 = Subtract(x=w1113, y=w1109) -> (x-y=w1112:dbl)
            "Time since lick" <- w1112
            n173 = shared-variable "My Computer\\michelle_library.lvlib\\Time_since_lick"(w1112) -> ()  [unwired: 1 in, 1 out]
          }
        }
        n174 = local read "Stop"() -> (w1096:bool)
      }
      n175 = while {
        stop <- w512 stop-if-true
        n176 = local read "LickBurst"() -> (w510:bool)
        n177 = Wait (ms)(milliseconds to wait=u32 10) -> ()  [unwired: 1 out]
        n178 = case shown="True" w510 {
          frame False {
          }
          frame True {
            n179 = flat-sequence {
              frame #0 {
                n180 = while {
                  stop <- w515 stop-if-true
                  n181 = local read "Time since lick"() -> (w516:dbl)
                  n182 = local read "BurstCriteria"() -> (w517:dbl)
                  n183 = Subtract(x=w516, y=w517) -> (x-y=w513:dbl)
                  n184 = Greater?(x=w513, y=0.0) -> (0:w515:bool)
                }
              }
              frame #1 {
                n185 = local write "LickBurst"(FALSE) -> ()
              }
            }
          }
        }
        n186 = shared-variable "My Computer\\michelle_library.lvlib\\Stop"() -> (w512:bool)  [unwired: 1 in, 1 out]
      }
      n187 = while {
        tunnel: w340 -> [w1233]
        stop <- w1231 stop-if-true
        n188 = local read "EntTS"() -> (w1223:dbl[][])
        n189 = local read "VidTS"() -> (w1222:dbl[][])
        n190 = Tick Count (ms)() -> (millisecond timer value=w1234:u32)
        n191 = Wait (ms)(milliseconds to wait=u32 10) -> ()  [unwired: 1 out]
        n192 = local read "ConsTS"() -> (w1226:dbl[][])
        n193 = Subtract(x=w1234, y=w1233) -> (x-y=w1230:u32)
        n194 = local read "RewTS"() -> (w1225:dbl[][])
        n195 = local read "LickTS"() -> (w1227:dbl[][])
        n196 = Divide(x=w1230, y=u32 1000) -> (x/y=→"Time":dbl)
        n197 = Build Array (concatenate) ("Build Matrix")(w1227, w1226, w1225, w1223, w1222) -> (w1224:T1)
        n198 = shared-variable "My Computer\\michelle_library.lvlib\\TSLog_Behavior"(w1224) -> ()  [unwired: 1 in, 1 out]
        n199 = local read "Stop"() -> (w1231:bool)
      }
      n200 = while {
        shift-right: [w654] -> _
        shift-left: _ -> [w655]
        stop <- w658 stop-if-true
        n201 = local read "Watch_Display"() -> (w657:bool)
        n202 = case shown="True" w657 {
          tunnel: w655 -> [w659 w661]
          tunnel: [w659 w660] -> w654
          frame False {
          }
          frame True {
            n203 = shared-variable "My Computer\\michelle_library.lvlib\\Display"() -> (w663:bool)  [unwired: 1 in, 1 out]
            n204 = local write "Misses"(0) -> ()
            n205 = case shown="False" w663 {
              tunnel: w661 -> [w666 w706]
              tunnel: [w664 w706] -> w660
              frame False {
                n206 = flat-sequence {
                  tunnel: w666 -> [w670]
                  tunnel: [w669] -> w665
                  tunnel: w665 -> [w696]
                  tunnel: [w695] -> w664
                  frame #0 {
                    n207 = while {
                      stop <- w685 stop-if-true
                      w686 = 10
                      n208 = local read "Its"() -> (w690:i32)
                      n209 = Wait (ms)(milliseconds to wait=w686) -> ()  [unwired: 1 out]
                      n210 = Increment(x=w690) -> (x+1=w689:i32)
                      n211 = local read "Consumption_Period"() -> (w683:i32)
                      n212 = local write "Its"(w689) -> ()
                      n213 = local read "Its"() -> (w687:i32)
                      n214 = local read "LickBurst"() -> (w691:bool)
                      n215 = Multiply(x=w687, y=w686) -> (x*y=w684:i32)
                      n216 = Greater?(x=w684, y=w683) -> (0:w682:bool)
                      n217 = Not(x=w691) -> (.not. x?=w688:bool)
                      n218 = Or(x=w688, y=w682) -> (x .or. y?=w685:bool)
                    }
                    n219 = Get Date/Time In Seconds() -> (seconds since 1Jan1904=w675:timestamp)
                    n220 = local write "Time_out"(FALSE) -> ()
                    n221 = shared-variable "My Computer\\michelle_library.lvlib\\Timeout"(FALSE) -> ()  [unwired: 1 in, 1 out]
                    n222 = local write "Active Trial"(FALSE) -> ()
                    n223 = shared-variable "My Computer\\michelle_library.lvlib\\ConsumptionON"(TRUE) -> ()  [unwired: 1 in, 1 out]
                    n224 = local read "TestTime"() -> (w672:dbl)
                    n225 = To Double Precision Float(number=w675) -> (double precision float=w673:dbl)
                    n226 = shared-variable "My Computer\\michelle_library.lvlib\\GlobalTime"() -> (w668:dbl)  [unwired: 1 in, 1 out]
                    n227 = Subtract(x=w673, y=w672) -> (x-y=w676:dbl)
                    n228 = shared-variable "My Computer\\michelle_library.lvlib\\Frame_clock"() -> (w667:u32)  [unwired: 1 in, 1 out]
                    n229 = Build Array(221, w676, w668, w667) -> (w671:T1)
                    n230 = Build Array (concatenate) ("Build Matrix")(w670, w671) -> (w669:T1)
                    n231 = local write "ConsTS"(w669) -> ()
                    "ConsumptionGo" <- TRUE
                  }
                  frame #1 {
                    n232 = Get Date/Time In Seconds() -> (seconds since 1Jan1904=w700:timestamp)
                    n233 = shared-variable "My Computer\\michelle_library.lvlib\\ConsumptionON"(FALSE) -> ()  [unwired: 1 in, 1 out]
                    n234 = local write "ConsumptionGo"(FALSE ("ConsumptionGo")) -> ()
                    n235 = local write "Watch_Display"(FALSE ("Watch_Display")) -> ()
                    n236 = local read "TestTime"() -> (w697:dbl)
                    n237 = To Double Precision Float(number=w700) -> (double precision float=w698:dbl)
                    n238 = shared-variable "My Computer\\michelle_library.lvlib\\GlobalTime"() -> (w693:dbl)  [unwired: 1 in, 1 out]
                    n239 = Subtract(x=w698, y=w697) -> (x-y=w701:dbl)
                    n240 = shared-variable "My Computer\\michelle_library.lvlib\\Frame_clock"() -> (w692:u32)  [unwired: 1 in, 1 out]
                    n241 = Build Array(222, w701, w693, w692) -> (w694:T1)
                    n242 = Build Array (concatenate) ("Build Matrix")(w696, w694) -> (w695:T1)
                    n243 = local write "Its"(0) -> ()
                    n244 = local write "ConsTS"(w695) -> ()
                  }
                }
              }
              frame True {
              }
            }
          }
        }
        n245 = Wait (ms)(milliseconds to wait=u32 5) -> ()  [unwired: 1 out]
        n246 = shared-variable "My Computer\\michelle_library.lvlib\\Stop"() -> (w658:bool)  [unwired: 1 in, 1 out]
      }
      n247 = flat-sequence {
        frame #0 {
          n248 = while {
            stop <- w722 stop-if-true
            n249 = shared-variable "My Computer\\michelle_library.lvlib\\Stim_loaded"() -> (w722:bool)  [unwired: 1 in, 1 out]
            "Stimuli Loaded" <- w722
          }
          n250 = Wait (ms)(milliseconds to wait=u32 10) -> ()  [unwired: 1 out]
        }
        frame #1 {
          n251 = Get Date/Time In Seconds() -> (seconds since 1Jan1904=w728:timestamp)
          n252 = local read "TestTime"() -> (w727:dbl)
          n253 = To Double Precision Float(number=w728) -> (double precision float=w726:dbl)
          n254 = shared-variable "My Computer\\michelle_library.lvlib\\InitiatedLag"() -> (w725:dbl)  [unwired: 1 in, 1 out]
          n255 = Subtract(x=w726, y=w727) -> (x-y=w723:dbl)
          n256 = Subtract(x=w723, y=w725) -> (x-y=→"Lag2":dbl)
        }
        frame #2 {
          n257 = local read "TestTime"() -> (w729:dbl)
          n258 = local read "Lag2"() -> (w730:dbl)
          n259 = Add(x=w729, y=w730) -> (x+y=w731:dbl)
          n260 = local write "TestTime"(w731) -> ()
        }
        frame #3 {
          n261 = shared-variable "My Computer\\michelle_library.lvlib\\Timings"() -> (→"Timings":dbl[])  [unwired: 1 in, 1 out]
          n262 = shared-variable "My Computer\\michelle_library.lvlib\\Stim_ID"() -> (→"Stim_ID":dbl[])  [unwired: 1 in, 1 out]
          n263 = Wait (ms)(milliseconds to wait=u32 10) -> ()  [unwired: 1 out]
          n264 = shared-variable "My Computer\\michelle_library.lvlib\\Reward_mat"() -> (→"Reward_mat":dbl[])  [unwired: 1 in, 1 out]
          n265 = shared-variable "My Computer\\michelle_library.lvlib\\Num_trials"() -> (w735:u32)  [unwired: 1 in, 1 out]
          n266 = Initialize Array(0.0 ("element"), w735) -> (→"Rewarded trials":dbl[])
        }
        frame #4 {
          n267 = while {
            shift-right: [w851] -> _
            shift-left: _ -> [w849]
            shift-right: [w847] -> _
            shift-left: _ -> [w846]
            shift-right: [w841] -> _
            shift-left: _ -> [w839]
            stop <- w852 stop-if-true
            n268 = local read "ConsumptionGo"() -> (w841:bool)
            n269 = shared-variable "My Computer\\michelle_library.lvlib\\Display"() -> (w847:bool)  [unwired: 1 in, 1 out]
            n270 = local read "Time_out"() -> (w851:bool)
            n271 = Wait (ms)(milliseconds to wait=u32 10) -> ()  [unwired: 1 out]
            n272 = Not(x=w851) -> (.not. x?=w850:bool)
            n273 = Not(x=w847) -> (.not. x?=w845:bool)
            n274 = Not(x=w841) -> (.not. x?=w842:bool)
            n275 = And(x=w850, y=w849) -> (x .and. y?=w844:bool)
            n276 = And(x=w846, y=w845) -> (x .and. y?=w840:bool)
            n277 = local read "Time_out"() -> (w848:bool)
            n278 = And(x=w839, y=w842) -> (x .and. y?=w838:bool)
            n279 = Or(x=w844, y=w840) -> (x .or. y?=w837:bool)
            n280 = Or(x=w837, y=w838) -> (x .or. y?=w836:bool)
            n281 = case shown="True" w836 {
              tunnel: w848 -> [w853 _]
              frame False {
                n282 = case shown="False" w853 {
                  frame False {
                    n283 = local read "ISI start time"() -> (w856:dbl)
                    n284 = local read "Time"() -> (w855:dbl)
                    n285 = Subtract(x=w855, y=w856) -> (x-y=w854:dbl)
                    n286 = shared-variable "My Computer\\michelle_library.lvlib\\ISI"(w854) -> ()  [unwired: 1 in, 1 out]
                    n287 = local write "ISI"(w854) -> ()
                  }
                  frame True {
                    n288 = local read "Time"() -> (w861:dbl)
                    n289 = Subtract(x=w861, y=0.11) -> (x-y=w858:dbl)
                    n290 = local write "ISI start time"(w858) -> ()
                    n291 = local read "Time"() -> (w859:dbl)
                    n292 = Subtract(x=w859, y=w858) -> (x-y=w857:dbl)
                    n293 = shared-variable "My Computer\\michelle_library.lvlib\\ISI"(w857) -> ()  [unwired: 1 in, 1 out]
                    n294 = local write "ISI"(w857) -> ()
                  }
                }
              }
              frame True {
                n295 = local read "Time"() -> (w866:dbl)
                n296 = Subtract(x=w866, y=0.11) -> (x-y=w863:dbl)
                "ISI start time" <- w863
                n297 = local read "Time"() -> (w864:dbl)
                n298 = Subtract(x=w864, y=w863) -> (x-y=w862:dbl)
                "ISI" <- w862
                n299 = shared-variable "My Computer\\michelle_library.lvlib\\ISI"(w862) -> ()  [unwired: 1 in, 1 out]
              }
            }
            n300 = local read "Stop"() -> (w852:bool)
          }
          n301 = while {
            stop <- w741 stop-if-true
            n302 = local read "Active Trial"() -> (w740:bool)
            n303 = case shown="True" w740 {
              frame False {
              }
              frame True {
                n304 = local write "Time_out"(FALSE) -> ()
                n305 = shared-variable "My Computer\\michelle_library.lvlib\\Timeout"(FALSE) -> ()  [unwired: 1 in, 1 out]
              }
            }
            n306 = Wait (ms)(milliseconds to wait=5) -> ()  [unwired: 1 out]
            n307 = shared-variable "My Computer\\michelle_library.lvlib\\Stop"() -> (w741:bool)  [unwired: 1 in, 1 out]
          }
          n308 = while {
            stop <- w762 stop-if-true
            n309 = shared-variable "My Computer\\michelle_library.lvlib\\Trial"() -> (w752:u32)  [unwired: 1 in, 1 out]
            n310 = Wait (ms)(milliseconds to wait=u32 10) -> ()  [unwired: 1 out]
            n311 = local read "Timings"() -> (w754:dbl[])
            n312 = local read "Time since lick"() -> (w761:dbl)
            n313 = Decrement(x=w752) -> (x-1=w751:u32)
            n314 = Index Array(array=w754, index=w751) -> (element=w753:dbl)
            n315 = Less?(x=w761, y=w753) -> (x < y?=w760:bool)
            n316 = shared-variable "My Computer\\michelle_library.lvlib\\Display"() -> (w757:bool)  [unwired: 1 in, 1 out]
            n317 = local read "ConsumptionGo"() -> (w749:bool)
            n318 = local read "Lick"() -> (w759:bool)
            n319 = And(x=w759, y=w760) -> (x .and. y?=w755:bool)
            n320 = Not(x=w757) -> (.not. x?=w756:bool)
            n321 = local read "Active Trial"() -> (w744:bool)
            n322 = And(x=w756, y=w755) -> (x .and. y?=w748:bool)
            n323 = Not(x=w749) -> (.not. x?=w750:bool)
            n324 = And(x=w748, y=w750) -> (x .and. y?=w746:bool)
            n325 = Not(x=w744) -> (.not. x?=w747:bool)
            n326 = And(x=w746, y=w747) -> (x .and. y?=w745:bool)
            n327 = case shown="True" w745 {
              frame False {
              }
              frame True {
                n328 = flat-sequence {
                  frame #0 {
                    w763 = TRUE
                    n329 = local read "TimeOutDuration"() -> (w764:i32)
                    n330 = xnode "DisplayOn 3"("C/DIO3 (DIO3)"=w763) -> ()  [unwired: 1 in, 1 out]
                    n331 = shared-variable "My Computer\\michelle_library.lvlib\\Timeout"(w763) -> ()  [unwired: 1 in, 1 out]
                    n332 = Wait (ms)(milliseconds to wait=w764) -> ()  [unwired: 1 out]
                    "Time_out" <- w763
                  }
                  frame #1 {
                    w800 = FALSE ("Timeout")
                    n333 = xnode "DisplayOn 4"("C/DIO3 (DIO3)"=w800) -> ()  [unwired: 1 in, 1 out]
                    n334 = local write "Time_out"(w800) -> ()
                    n335 = shared-variable "My Computer\\michelle_library.lvlib\\Timeout"(w800) -> ()  [unwired: 1 in, 1 out]
                  }
                }
              }
            }
            n336 = local read "Stop"() -> (w762:bool)
          }
          n337 = while {
            shift-right: [w913] -> _
            shift-left: _ -> [w912]
            shift-right: [w905] -> _
            shift-left: _ -> [w906]
            stop <- w915 stop-if-true
            n338 = local read "Active Trial"() -> (w910:bool)
            n339 = Wait (ms)(milliseconds to wait=u32 10) -> ()  [unwired: 1 out]
            n340 = local read "Lick"() -> (w911:bool)
            n341 = And(x=w910, y=w911) -> (x .and. y?=w909:bool)
            n342 = Or(x="Give reward", y=w909) -> (x .or. y?=w908:bool)
            n343 = case shown="True" w908 {
              tunnel: [w917 w924] -> w913
              tunnel: w912 -> [w917 w923]
              tunnel: w906 -> [w916 w921]
              tunnel: [w916 w920] -> w905
              frame False {
              }
              frame True {
                n344 = flat-sequence {
                  tunnel: w921 -> [w930]
                  tunnel: [w927] -> w918
                  tunnel: [w986] -> w919
                  tunnel: w918 -> [w984]
                  tunnel: [w1030] -> w920
                  tunnel: w919 -> [w1030]
                  frame #0 {
                    w945 = TRUE ("C/DIO0 (DIO0)")
                    n345 = Get Date/Time In Seconds() -> (seconds since 1Jan1904=w934:timestamp)
                    n346 = local write "Time_out"(FALSE) -> ()
                    n347 = shared-variable "My Computer\\michelle_library.lvlib\\Timeout"(FALSE) -> ()  [unwired: 1 in, 1 out]
                    n348 = local write "GoAhead"(FALSE) -> ()
                    n349 = Wait (ms)(milliseconds to wait=u32 100) -> ()  [unwired: 1 out]
                    n350 = local read "TestTime"() -> (w928:dbl)
                    n351 = shared-variable "My Computer\\michelle_library.lvlib\\Trial"() -> (w944:u32)  [unwired: 1 in, 1 out]
                    n352 = shared-variable "My Computer\\michelle_library.lvlib\\GlobalReward"() -> (w936:dbl)  [unwired: 1 in, 1 out]
                    n353 = To Double Precision Float(number=w934) -> (double precision float=w933:dbl)
                    n354 = shared-variable "My Computer\\michelle_library.lvlib\\GlobalTime"() -> (w926:dbl)  [unwired: 1 in, 1 out]
                    n355 = local read "Rewarded trials"() -> (w942:dbl[])
                    n356 = Subtract(x=w933, y=w928) -> (x-y=w932:dbl)
                    n357 = xnode "Reward 3"("C/DIO0 (DIO0)"=w945) -> ()  [unwired: 1 in, 1 out]
                    n358 = Decrement(x=w944) -> (x-1=w943:u32)
                    n359 = shared-variable "My Computer\\michelle_library.lvlib\\Frame_clock"() -> (w925:u32)  [unwired: 1 in, 1 out]
                    n360 = Increment(x=w936) -> (x+1=w935:dbl)
                    n361 = Replace Array Subset(array=w942, new element=1.0 ("new element/subarray"), index=w943) -> (w940:dbl[])
                    n362 = Build Array(551, w932, w926, w925) -> (w931:T1)
                    n363 = local write "Rewarded trials"(w940) -> ()
                    n364 = shared-variable "My Computer\\michelle_library.lvlib\\GlobalReward"(w935) -> ()  [unwired: 1 in, 1 out]
                    n365 = Build Array (concatenate) ("Build Matrix")(w930, w931) -> (w927:T1)
                    n366 = local write "RewTS"(w927) -> ()
                    "Reward" <- w945
                    "Watch_Display" <- w945
                  }
                  frame #1 {
                    w994 = FALSE ("C/DIO0 (DIO0)")
                    n367 = Get Date/Time In Seconds() -> (seconds since 1Jan1904=w991:timestamp)
                    n368 = local read "TestTime"() -> (w985:dbl)
                    n369 = local write "Give reward"(FALSE ("Give reward")) -> ()
                    n370 = Wait (ms)(milliseconds to wait=u32 20) -> ()  [unwired: 1 out]
                    n371 = shared-variable "My Computer\\michelle_library.lvlib\\GlobalTime"() -> (w983:dbl)  [unwired: 1 in, 1 out]
                    n372 = To Double Precision Float(number=w991) -> (double precision float=w990:dbl)
                    n373 = xnode "Reward 4"("C/DIO0 (DIO0)"=w994) -> ()  [unwired: 1 in, 1 out]
                    n374 = local write "Reward"(w994) -> ()
                    n375 = Subtract(x=w990, y=w985) -> (x-y=w989:dbl)
                    n376 = shared-variable "My Computer\\michelle_library.lvlib\\Frame_clock"() -> (w982:u32)  [unwired: 1 in, 1 out]
                    n377 = Build Array(552, w989, w983, w982) -> (w987:T1)
                    n378 = Build Array (concatenate) ("Build Matrix")(w984, w987) -> (w986:T1)
                    n379 = local write "RewTS"(w986) -> ()
                  }
                  frame #2 {
                    n380 = Wait (ms)(milliseconds to wait=u32 50) -> ()  [unwired: 1 out]
                  }
                }
                n381 = Increment(x=w923) -> (x+1=w924:u16)
                "Rewards" <- w924
                n382 = local write "Active Trial"(FALSE ("Active Trial")) -> ()
              }
            }
            n383 = local read "Stop"() -> (w915:bool)
          }
          n384 = while {
            stop <- w880 stop-if-true
            n385 = shared-variable "My Computer\\michelle_library.lvlib\\Trial"() -> (w876:u32)  [unwired: 1 in, 1 out]
            n386 = shared-variable "My Computer\\michelle_library.lvlib\\Trial"() -> (w872:u32)  [unwired: 1 in, 1 out]
            n387 = Wait (ms)(milliseconds to wait=u32 10) -> ()  [unwired: 1 out]
            n388 = local read "Rewarded trials"() -> (w873:dbl[])
            n389 = local read "Reward_mat"() -> (w875:dbl[])
            n390 = Decrement(x=w876) -> (x-1=w877:u32)
            n391 = Decrement(x=w872) -> (x-1=w871:u32)
            n392 = Index Array(array=w875, index=w877) -> (element=w878:dbl)
            n393 = Index Array(array=w873, index=w871) -> (element=w870:dbl)
            n394 = Equal To 0?(x=w870) -> (x = 0?=w869:bool)
            n395 = Equal?(x=w878, y=1.0) -> (x = y?=w868:bool)
            n396 = And(x=w868, y=w869) -> (x .and. y?=w867:bool)
            n397 = case shown="True" w867 {
              frame False {
                n398 = local write "Active Trial"(FALSE ("Active_trial")) -> ()
              }
              frame True {
                n399 = shared-variable "My Computer\\michelle_library.lvlib\\Trial"() -> (w883:u32)  [unwired: 1 in, 1 out]
                n400 = local read "Stim_ID"() -> (w885:dbl[])
                n401 = Decrement(x=w883) -> (x-1=w884:u32)
                n402 = Index Array(array=w885, index=w884) -> (element=w882:dbl)
                n403 = case shown="1, Default" w882 {
                  frame 1, Default {
                    n404 = shared-variable "My Computer\\michelle_library.lvlib\\ISI_Time"() -> (w891:dbl)  [unwired: 1 in, 1 out]
                    n405 = local read "ActiveTime"() -> (w886:dbl)
                    n406 = Less?(x=w891, y=w886) -> (x < y?=w889:bool)
                    n407 = Greater?(x=w891, y=0.1) -> (0:w888:bool)
                    n408 = And(x=w889, y=w888) -> (x .and. y?=w887:bool)
                    n409 = case shown="True" w887 {
                      frame False {
                        n410 = local write "Active Trial"(FALSE ("Active Trial")) -> ()
                      }
                      frame True {
                        n411 = local read "Time"() -> (w895:dbl)
                        n412 = local write "Active Trial"(TRUE ("Active Trial")) -> ()
                        n413 = Add(x=w895, y=-0.11) -> (x+y=w893:dbl)
                        n414 = local write "Time of last lick"(w893) -> ()
                      }
                    }
                  }
                  frame 2 {
                    n415 = shared-variable "My Computer\\michelle_library.lvlib\\ISI_Time"() -> (w901:dbl)  [unwired: 1 in, 1 out]
                    n416 = local read "ActiveTime"() -> (w897:dbl)
                    n417 = Less?(x=w901, y=w897) -> (x < y?=w899:bool)
                    n418 = Greater?(x=w901, y=0.1) -> (0:w900:bool)
                    n419 = And(x=w900, y=w899) -> (x .and. y?=w898:bool)
                    n420 = case shown="True" w898 {
                      frame False {
                        n421 = local write "Active Trial"(FALSE ("Active Trial")) -> ()
                      }
                      frame True {
                        "Active Trial" <- TRUE ("Active Trial")
                      }
                    }
                  }
                }
              }
            }
            n422 = local read "Stop"() -> (w880:bool)
          }
        }
      }
      n423 = while {
        shift-right: [w344] -> _
        shift-left: _ -> [w343]
        stop <- w342 stop-if-true
        n424 = xnode "Analog input (1 sample)"() -> ("C/AI0 (AI0)"=w341:dbl)  [unwired: 1 in, 1 out]
        n425 = Wait (ms)(milliseconds to wait=u32 10) -> ()  [unwired: 1 out]
        n426 = Build Array (concatenate)(w343, w341) -> (w344:dbl[])
        "LightPlot" <- w344
        "LightArray" <- w344
        n427 = local write "Light"(w341) -> ()
        n428 = local read "Stop"() -> (w342:bool)
      }
      n429 = flat-sequence {
        frame #0 {
          n430 = xnode "Encoder 4"("Reset Counter"=TRUE) -> ()  [unwired: 1 in, 4 out]
        }
        frame #1 {
          n431 = while {
            shift-right: [w436] -> _
            shift-left: _ -> [w437]
            stop <- w441 stop-if-true
            n432 = local read "GetVidFrame"() -> (w431:i32)
            n433 = local read "VidFrameClock"() -> (w435:i32)
            n434 = Equal?(x=w435, y=1) -> (x = y?=w434:bool)
            n435 = Equal?(x=w431, y=1) -> (x = y?=w430:bool)
            n436 = And(x=w434, y=w430) -> (x .and. y?=w433:bool)
            n437 = case shown="True" w433 {
              tunnel: w437 -> [w445 w448]
              tunnel: [w445 w447] -> w436
              frame False {
              }
              frame True {
                n438 = local read "TestTime"() -> (w454:dbl)
                n439 = shared-variable "My Computer\\michelle_library.lvlib\\GlobalTime"() -> (w451:dbl)  [unwired: 1 in, 1 out]
                n440 = Get Date/Time In Seconds() -> (seconds since 1Jan1904=w456:timestamp)
                n441 = shared-variable "My Computer\\michelle_library.lvlib\\Frame_clock"() -> (w452:u32)  [unwired: 1 in, 1 out]
                n442 = To Double Precision Float(number=w456) -> (double precision float=w455:dbl)
                n443 = Subtract(x=w455, y=w454) -> (x-y=w453:dbl)
                n444 = Build Array(881, w453, w451, w452) -> (w450:T1)
                n445 = Build Array (concatenate) ("Build Matrix")(w448, w450) -> (w447:T1)
                n446 = local write "GetVidFrame"(0) -> ()
                n447 = local write "VidTS"(w447) -> ()
              }
            }
            n448 = xnode "Encoder 3"() -> ("Counter Value"=w443:i32)  [unwired: 2 in, 3 out]
            n449 = Multiply(x=w443, y=-1) -> (x*y=w440:i32)
            "VidFrameClock" <- w440
            n450 = Equal?(x=w440, y=720000) -> (x = y?=w441:bool)
            n451 = shared-variable "My Computer\\michelle_library.lvlib\\VidFrameClock1"(w440) -> ()  [unwired: 1 in, 1 out]
            n452 = local write "Stop"(w441) -> ()
            n453 = Wait (ms)(milliseconds to wait=u32 1) -> ()  [unwired: 1 out]
          }
        }
        frame #2 {
          n454 = local read "Stop"() -> (w503:bool)
          n455 = shared-variable "My Computer\\michelle_library.lvlib\\Stop"(w503) -> ()  [unwired: 1 in, 1 out]
        }
      }
    }
  }
